vi "test-quintic-spline-06.vi"() -> (3 "Test Passed":bool)   [LabVIEW 2019]
uses:
  <vilib>/Rock Robotics/WPI/ThirdParty/JAS_Junk/TrajLib/POSEwCURVATURE.ctl
  <vilib>/Rock Robotics/WPI/ThirdParty/JAS_Junk/TrajLib/POSE2D.ctl
  <vilib>/Rock Robotics/WPI/ThirdParty/JAS_Junk/TrajLib/TRANSLATION2D.ctl
  <vilib>/Rock Robotics/WPI/ThirdParty/JAS_Junk/TrajLib/ROTATION2D.ctl
  <vilib>/Rock Robotics/WPI/ThirdParty/JAS_Junk/TrajLib/Rotation_CreateAngle.vi
  <vilib>/Rock Robotics/WPI/ThirdParty/JAS_Junk/TrajLib/Translation_Create.vi
  <vilib>/Rock Robotics/WPI/ThirdParty/JAS_Junk/TrajLib/Util_CalcDist.vi
  <vilib>/Rock Robotics/WPI/ThirdParty/JAS_Junk/TrajLib/Trajectory_Library.lvlib
panel:
  out "XY Graph":cluster{dbl[], dbl[]}(graph)
  out "Numb\nWaypoints":i32
  out "All Interior \nwayPoints\nFound (True)":bool
  out "end rot = 0":dbl
  out "end y = 0":dbl
  out "end x = 0":dbl
  out "start rot = 0":dbl
  out "start y = 0":dbl
  out "start x = 0":dbl
  out "max dtheta < 0.0872":dbl
  out "max dy < 0.00127":dbl
  out "max dx  < 0.127":dbl
  out "Overall Error":errorcluster
  out "Elements":i32
  out "Create Spline Error":errorcluster
  out "SplinePoses\nWCurve":T1[](array[typedef]) {"POSE"."ROTATION"."SIN" format="%13.4f"; "POSE"."ROTATION"."COS" format="%13.4f"; "POSE"."ROTATION"."VALUE" format="%13.4f"; "POSE"."TRANSLATION"."Y" format="%14.3f"; "POSE"."TRANSLATION"."X" format="%14.3f"}
  out "Elapsed Time":dbl
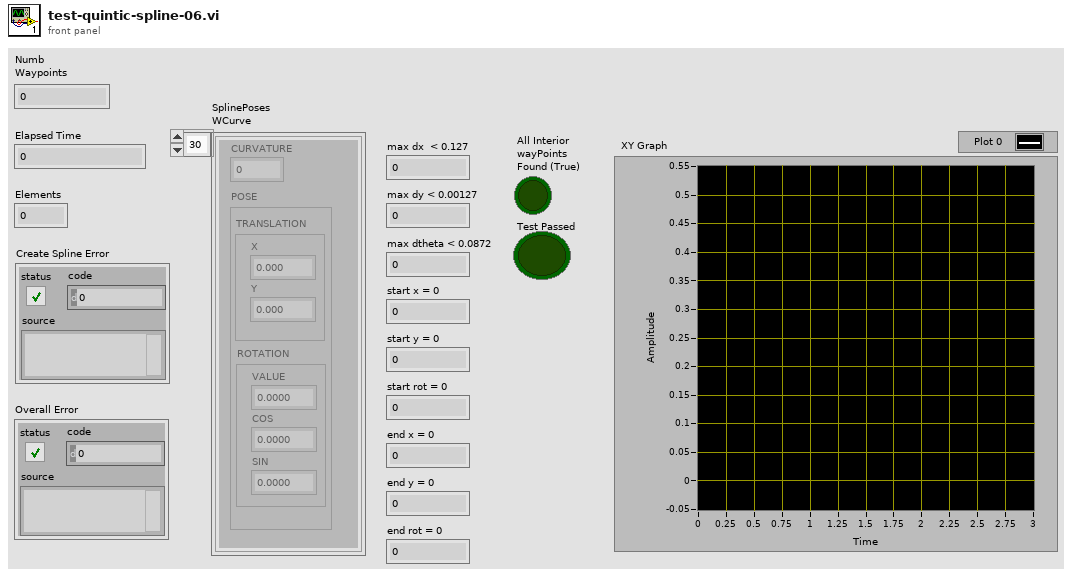
[diagram p1: front panel]
types:
  T1 = typedef "Trajectory_Library.lvlib/POSEwCURVATURE.ctl" = cluster{"CURVATURE":dbl, "POSE":T2}
  T2 = typedef "Trajectory_Library.lvlib/POSE2D.ctl" = cluster{"TRANSLATION":T3, "ROTATION":T4}
  T3 = typedef "Trajectory_Library.lvlib/TRANSLATION2D.ctl" = cluster{"X":dbl, "Y":dbl}
  T4 = typedef "Trajectory_Library.lvlib/ROTATION2D.ctl" = cluster{"VALUE":dbl, "COS":dbl, "SIN":dbl}
  T5 = typedef "Trajectory_Library.lvlib/SPLINE_CTRL_VECTOR.ctl" = cluster{"Xs":dbl[], "Ys":dbl[]}
  T6 = typedef "Trajectory_Library.lvlib/SPLINE.ctl" = cluster{"Degree":i32, "Coefficients":T7}
  T7 = typedef "NI_Matrix.lvlib/RealMatrix.ctl" = dbl[][]
  T8 = typedef "Trajectory_Library.lvlib/TWIST2D.ctl" = cluster{"dX":dbl, "dY":dbl, "dTHETA":dbl}
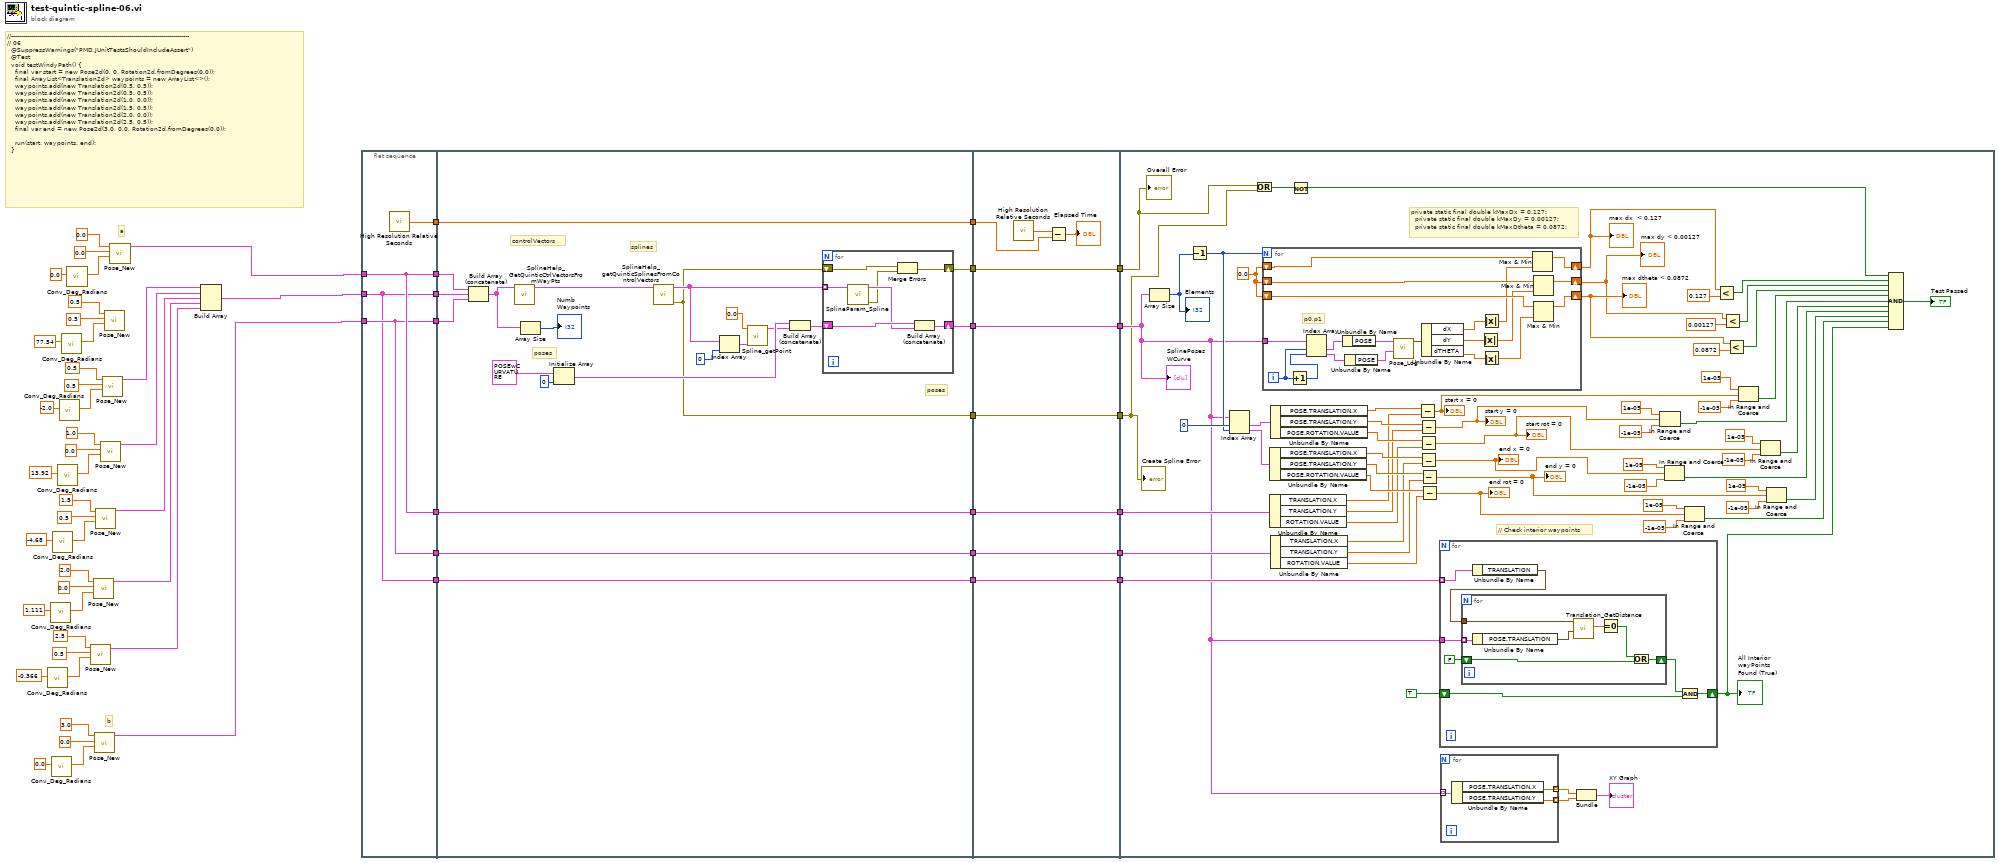
[diagram p0: block diagram]
diagram:
  # "b"
  # "a"
  # "//-----------------------------------------------------------------------------------------\n// 06\n  @SuppressWarnings(\"PMD.JUnitTestsShouldIncludeAssert\")\n  @Test\n  void testWindyPath() {\n    final var start = new Pose2d(0, 0, Rotation2d.fromDegrees(0.0));\n    final ArrayList<Translation2d> waypoints = new ArrayList<>();\n    waypoints.add(new Translation2d(0.5, 0.5));\n    waypoints.add(new Translation2d(0.5, 0.5));\n    waypoints.add(new Translation2d(1.0, 0.0));\n    waypoints.add(new Translation2d(1.5, 0.5));\n    waypoints.add(new Translation2d(2.0, 0.0));\n    waypoints.add(new Translation2d(2.5, 0.5));\n    final var end = new Pose2d(3.0, 0.0, Rotation2d.fromDegrees(0.0));\n\n    run(start, waypoints, end);\n  }"
  n1 = call <vilib>:"Conv_Deg_Radians.vi"("Degress"=-0.366) -> ("Radians"=w10:dbl)  [unwired: 10 in]
  n2 = call <vilib>:"Conv_Deg_Radians.vi"("Degress"=1.111) -> ("Radians"=w14:dbl)  [unwired: 10 in]
  n3 = call <vilib>:"Conv_Deg_Radians.vi"("Degress"=0.0) -> ("Radians"=w38:dbl)  [unwired: 10 in]
  n4 = call <vilib>:"Conv_Deg_Radians.vi"("Degress"=-4.68) -> ("Radians"=w18:dbl)  [unwired: 10 in]
  n5 = call <vilib>:"Conv_Deg_Radians.vi"("Degress"=13.92) -> ("Radians"=w22:dbl)  [unwired: 10 in]
  n6 = call <vilib>:"Conv_Deg_Radians.vi"("Degress"=-2.0) -> ("Radians"=w26:dbl)  [unwired: 10 in]
  n7 = call <vilib>:"Conv_Deg_Radians.vi"("Degress"=77.54) -> ("Radians"=w30:dbl)  [unwired: 10 in]
  n8 = call <vilib>:"Conv_Deg_Radians.vi"("Degress"=0.0) -> ("Radians"=w35:dbl)  [unwired: 10 in]
  n9 = call <vilib>:"Pose_New.vi"("Heading"=w10, "Y"=0.5, "X"=2.5) -> ("out POSe"=w4:T2)  [unwired: 8 in]
  n10 = call <vilib>:"Pose_New.vi"("Heading"=w14, "Y"=0.0, "X"=2.0) -> ("out POSe"=w5:T2)  [unwired: 8 in]
  n11 = call <vilib>:"Pose_New.vi"("Heading"=w38, "Y"=0.0, "X"=3.0) -> ("out POSe"=w1:T2)  [unwired: 8 in]
  n12 = call <vilib>:"Pose_New.vi"("Heading"=w18, "Y"=0.5, "X"=1.5) -> ("out POSe"=w6:T2)  [unwired: 8 in]
  n13 = call <vilib>:"Pose_New.vi"("Heading"=w22, "Y"=0.0, "X"=1.0) -> ("out POSe"=w7:T2)  [unwired: 8 in]
  n14 = call <vilib>:"Pose_New.vi"("Heading"=w26, "Y"=0.5, "X"=0.5) -> ("out POSe"=w8:T2)  [unwired: 8 in]
  n15 = call <vilib>:"Pose_New.vi"("Heading"=w30, "Y"=0.5, "X"=0.5) -> ()  [unwired: 8 in, 1 out]
  n16 = call <vilib>:"Pose_New.vi"("Heading"=w35, "Y"=0.0, "X"=0.0) -> ("out POSe"=w3:T2)  [unwired: 8 in]
  n17 = Build Array(w8, w7, w6, w5, w4) -> (w2:T2[])
  n18 = flat-sequence {
    tunnel: w3 -> [w63]
    tunnel: [w63] -> w60
    tunnel: w1 -> [w62]
    tunnel: [w62] -> w59
    tunnel: [w64] -> w58
    tunnel: [w63] -> w50
    tunnel: [w62] -> w47
    tunnel: [w61] -> w42
    tunnel: w2 -> [w61]
    tunnel: [w61] -> w41
    tunnel: w60 -> [w70]
    tunnel: w59 -> [w68]
    tunnel: [w86] -> w57
    tunnel: w58 -> [w86]
    tunnel: [w76] -> w56
    tunnel: [w75] -> w54
    tunnel: [w74] -> w52
    tunnel: w50 -> [w73]
    tunnel: [w73] -> w49
    tunnel: w47 -> [w72]
    tunnel: [w72] -> w46
    tunnel: [w71] -> w43
    tunnel: w42 -> [w71]
    tunnel: w41 -> [w65]
    tunnel: w57 -> [w102]
    tunnel: w56 -> [w101]
    tunnel: [w101] -> w55
    tunnel: w54 -> [w100]
    tunnel: [w100] -> w53
    tunnel: w52 -> [w99]
    tunnel: [w99] -> w51
    tunnel: w49 -> [w96]
    tunnel: [w96] -> w48
    tunnel: w46 -> [w95]
    tunnel: [w95] -> w45
    tunnel: [w94] -> w44
    tunnel: w43 -> [w94]
    tunnel: w55 -> [w143]
    tunnel: w53 -> [w131]
    tunnel: w51 -> [w130]
    tunnel: w48 -> [w165]
    tunnel: w45 -> [w164]
    tunnel: w44 -> [w147]
    frame #0 {
      n19 = call <vilib>:"High Resolution Relative Seconds.vi"() -> ("relative seconds"=w64:dbl)
    }
    frame #1 {
      # "poses"
      # "poses"
      # "splines"
      # "controlVectors"
      n20 = Build Array (concatenate)(w70, w65, w68) -> (w67:T2[])
      n21 = call <vilib>:"SplineHelp_GetQuinticCtrlVectorsFromWayPts.vi"("WayPoints"=w67) -> ("SplineControlVectors"=w69:T5[])  [unwired: 10 in]
      n22 = Array Size(array=w67) -> (size(s)=→"Numb\nWaypoints":i32)
      n23 = Initialize Array(T1 {"CURVATURE"=0.0, "POSE"={"TRANSLATION"={"X"=0.0, "Y"=0.0}, "ROTATION"={"VALUE"=0.0, "COS"=1.0, "SIN"=0.0}}} ("POSEwCURVATURE"), 0 ("dimension size")) -> (w80:T1[])
      n24 = call <vilib>:"SplineHelp_getQuinticSplinesFromControlVectors.vi"("ControlVectors"=w69) -> ("error out"=w75:errorcluster, "splines"=w77:T6[])  [unwired: 9 in]
      n25 = Index Array(array=w77, index=0) -> (element=w82:T6)
      n26 = call <vilib>:"Spline_getPoint.vi"("inputSPLINE"=w82, "Time"=0.0) -> ("POSEwCURVATURE"=w79:T1)  [unwired: 9 in]
      n27 = Build Array (concatenate)(w80, w79) -> (w78:T1[])
      n28 = for {
        shift-right: [w90] -> w76
        shift-left: w78 -> [w92]
        tunnel: w77 -> [w93] mode=indexing
        shift-right: [w88] -> w74
        shift-left: w75 -> [w89]
        n29 = call <vilib>:"SplineParam_Spline.vi"("inputSPLINE"=w93) -> ("error out"=w87:errorcluster, "outputPOSEwCURVATURE"=w91:T1[])  [unwired: 9 in]
        n30 = Merge Errors(w89, w87) -> (w88:errorcluster)
        n31 = Build Array (concatenate)(w92, w91) -> (w90:T1[])
      }
    }
    frame #2 {
      n32 = call <vilib>:"High Resolution Relative Seconds.vi"() -> ("relative seconds"=w97:dbl)
      n33 = Subtract(x=w97, y=w102) -> (x-y=→"Elapsed Time":dbl)
    }
    frame #3 {
      w166 = 0.0
      # "// Check interior waypoints"
      # "private static final double kMaxDx = 0.127;\n  private static final double kMaxDy = 0.00127;\n  private static final double kMaxDtheta = 0.0872;"
      n34 = Array Size(array=w143) -> (size(s)=w167:i32)
      "Elements" <- w167
      n35 = Decrement(x=w167) -> (x-1=w162:i32)
      n36 = Index Array(array=w143, index #1=0 ("index"), index #2=w162) -> (element #1=w161:T1, element #2=w160:T1)
      n37 = Or(x=w130, y=w131) -> (x .or. y?=w132:bool)
      n38 = for {
        N: w162 -> [_]
        tunnel: w143 -> [w202]
        shift-right: [w193] -> w136
        shift-left: w166 -> [w190]
        shift-right: [w191] -> w138
        shift-left: w166 -> [w188]
        shift-right: [w192] -> w137
        shift-left: w166 -> [w189]
        i -> [w204]
        # "p0,p1"
        n39 = Increment(x=w204) -> (x+1=w203:i32)
        n40 = Index Array(array=w202, index #1=w204, index #2=w203) -> (element #1=w201:T1, element #2=w200:T1)
        n41 = Unbundle By Name(w201) -> ("POSE"=w199:T2)
        n42 = Unbundle By Name(w200) -> ("POSE"=w198:T2)
        n43 = call <vilib>:"Pose_Log.vi"("end POSE"=w198, "in POSE"=w199) -> ("out TWIST"=w197:T8)  [unwired: 9 in]
        n44 = Unbundle By Name(w197) -> ("dX"=w194:dbl, "dY"=w195:dbl, "dTHETA"=w196:dbl)
        n45 = Absolute Value(x=w195) -> (abs(x)=w186:dbl)
        n46 = Absolute Value(x=w194) -> (abs(x)=w187:dbl)
        n47 = Absolute Value(x=w196) -> (abs(x)=w185:dbl)
        n48 = Max & Min(x=w190, y=w187) -> (max(x,y)=w193:dbl)  [unwired: 1 out]
        n49 = Max & Min(x=w189, y=w186) -> (max(x,y)=w192:dbl)  [unwired: 1 out]
        n50 = Max & Min(x=w188, y=w185) -> (max(x,y)=w191:dbl)  [unwired: 1 out]
      }
      "max dx  < 0.127" <- w136
      "max dy < 0.00127" <- w137
      "max dtheta < 0.0872" <- w138
      n51 = Unbundle By Name(w160) -> ("POSE.TRANSLATION.X"=w156:dbl, "POSE.TRANSLATION.Y"=w155:dbl, "POSE.ROTATION.VALUE"=w154:dbl)
      n52 = Unbundle By Name(w165) -> ("TRANSLATION.X"=w153:dbl, "TRANSLATION.Y"=w152:dbl, "ROTATION.VALUE"=w151:dbl)
      n53 = Unbundle By Name(w161) -> ("POSE.TRANSLATION.X"=w159:dbl, "POSE.TRANSLATION.Y"=w158:dbl, "POSE.ROTATION.VALUE"=w157:dbl)
      n54 = Unbundle By Name(w164) -> ("TRANSLATION.X"=w150:dbl, "TRANSLATION.Y"=w149:dbl, "ROTATION.VALUE"=w148:dbl)
      n55 = Not(x=w132) -> (.not. x?=w129:bool)
      n56 = Subtract(x=w159, y=w153) -> (x-y=w125:dbl)
      "start x = 0" <- w125
      n57 = Subtract(x=w158, y=w152) -> (x-y=w104:dbl)
      "start y = 0" <- w104
      n58 = Subtract(x=w157, y=w151) -> (x-y=w108:dbl)
      "start rot = 0" <- w108
      n59 = Subtract(x=w156, y=w150) -> (x-y=w109:dbl)
      "end x = 0" <- w109
      n60 = Subtract(x=w155, y=w149) -> (x-y=w116:dbl)
      "end y = 0" <- w116
      n61 = Subtract(x=w154, y=w148) -> (x-y=w120:dbl)
      "end rot = 0" <- w120
      n62 = for {
        tunnel: w147 -> [w172] mode=indexing
        tunnel: w143 -> [w177]
        shift-right: [w176] -> w128
        shift-left: TRUE -> [w175]
        n63 = Unbundle By Name(w172) -> ("TRANSLATION"=w171:T3)
        n64 = for {
          tunnel: w177 -> [w181] mode=indexing
          shift-right: [w184] -> w173
          shift-left: FALSE -> [w183]
          tunnel: w171 -> [w182]
          n65 = Unbundle By Name(w181) -> ("POSE.TRANSLATION"=w180:T3)
          n66 = call <vilib>:"Translation_GetDistance.vi"("other Translation"=w180, "In Translation"=w182) -> ("Distance"=w179:dbl)  [unwired: 9 in]
          n67 = Equal To 0?(x=w179) -> (x = 0?=w178:bool)
          n68 = Or(x=w178, y=w183) -> (x .or. y?=w184:bool)
        }
        n69 = And(x=w173, y=w175) -> (x .and. y?=w176:bool)
      }
      "All Interior \nwayPoints\nFound (True)" <- w128
      n70 = for {
        tunnel: [w170] -> w145 mode=indexing
        tunnel: [w169] -> w144 mode=indexing
        tunnel: w143 -> [w168] mode=indexing
        n71 = Unbundle By Name(w168) -> ("POSE.TRANSLATION.X"=w170:dbl, "POSE.TRANSLATION.Y"=w169:dbl)
      }
      n72 = Bundle(w145, w144) -> (→"XY Graph":cluster{dbl[], dbl[]})  [unwired: 1 in]
      n73 = In Range and Coerce(upper limit=1e-05, x=w104, lower limit=-1e-05) -> (In Range?=w105:bool)  [unwired: 1 out]
      n74 = In Range and Coerce(upper limit=1e-05, x=w109, lower limit=-1e-05) -> (In Range?=w111:bool)  [unwired: 1 out]
      n75 = In Range and Coerce(upper limit=1e-05, x=w120, lower limit=-1e-05) -> (In Range?=w121:bool)  [unwired: 1 out]
      n76 = Less?(x=w136, y=0.127) -> (x < y?=w135:bool)
      n77 = Less?(x=w137, y=0.00127) -> (x < y?=w134:bool)
      n78 = Less?(x=w138, y=0.0872) -> (x < y?=w133:bool)
      n79 = In Range and Coerce(upper limit=1e-05, x=w125, lower limit=-1e-05) -> (In Range?=w124:bool)  [unwired: 1 out]
      n80 = In Range and Coerce(upper limit=1e-05, x=w108, lower limit=-1e-05) -> (In Range?=w110:bool)  [unwired: 1 out]
      n81 = In Range and Coerce(upper limit=1e-05, x=w116, lower limit=-1e-05) -> (In Range?=w117:bool)  [unwired: 1 out]
      n82 = Compound Arithmetic op=AND(w129, w135, w134, w133, w124, w105, w110, w111, w117, w121, w128) -> (→"Test Passed":bool)
      "SplinePoses\nWCurve" <- w143
      "Create Spline Error" <- w131
      "Overall Error" <- w130
    }
  }
